vi "Dialog.vi"(11 "Status":string) -> (3 "Cancelled?":bool)   [LabVIEW 2019]
doc: "Use this template to create a dialog box with event handling."
panel:
  in  "OK":bool
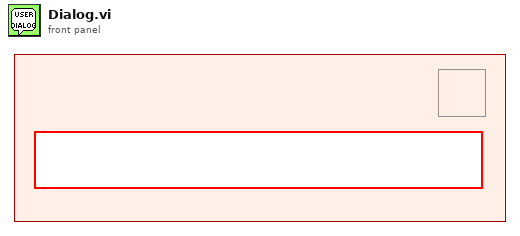
[diagram p1: front panel]
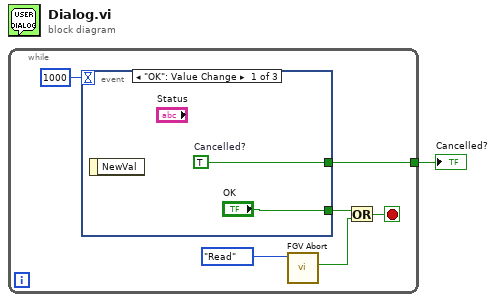
[diagram p0: block diagram]
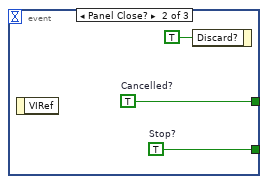
[diagram p2: hidden frame]
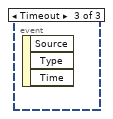
[diagram p3: hidden frame]
diagram:
  n1 = while {
    tunnel: [w7] -> w1
    stop <- w2 stop-if-true
    n2 = event shown="[0] \"OK\": Value Change" {
      selector: _ -> [_ _ _]
      dyn-events: _ -> [_ _ _]
      timeout: 1000 -> [_ _ _]
      tunnel: ["OK" w11 _] -> w3
      tunnel: [w9 w10 _] -> w7
      event "OK": Value Change {
        w9 = TRUE  # Cancelled?
        n3 = event-data() -> ()  [unwired: 1 in, 1 out]
      }
      event Panel Close? {
        w10 = TRUE  # Cancelled?
        w11 = TRUE  # Stop?
        n4 = event-data() -> ()  [unwired: 1 in, 1 out]
        n5 = event-data("Discard?"=TRUE) -> ()  [unwired: 1 in, 1 out]
      }
      event Timeout {
        n6 = event-data() -> ()  [unwired: 1 in, 3 out]
      }
    }
    n7 = call "FGV Abort.vi"("Action"=enum16{"Initialize", "Read", "Write"}."Read") -> ("Out"=w4:bool)  [unwired: 9 in, 1 out]
    n8 = Or(x=w3, y=w4) -> (x .or. y?=w2:bool)
  }
  "Cancelled?" <- w1
